vi "CheckCore.vi"(8 "error in (no error)":errorcluster, 9 "# of Refs":i32, 10 "References":refnum<vi>[](array[refnum]), 11 "Invoke in":refnum<class "Invoke.lvclass">) -> (0 "error out":errorcluster, 1 "Reject?":bool, 2 "dup References":refnum<vi>[](array[refnum]), 3 "Invoke out":refnum<class "Invoke.lvclass">)   [LabVIEW 2014, in "BuildSecurity.lvlib" / "Invoke.lvclass"]
doc: "Determines if any blacklisted invoke node exists in the VI."
uses:
  Invoke.lvclass
  Blacklist.lvclass/Blacklist.ctl
  ReadItems.vi
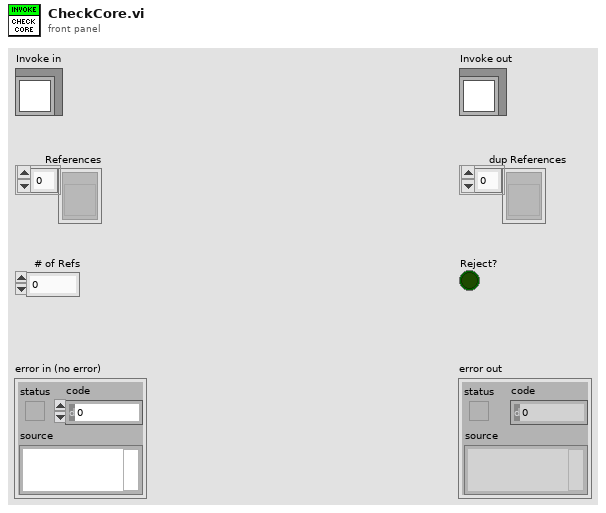
[diagram p1: front panel]
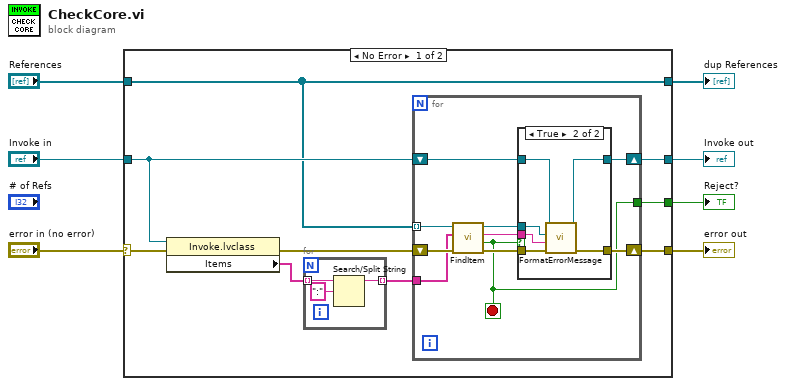
[diagram p0: block diagram]
diagram:
  n1 = case shown="No Error" "error in (no error)" {
    selector: "error in (no error)" -> [w16 w40]
    tunnel: "Invoke in" -> [w13 w39]
    tunnel: [w10 w40] -> w5
    tunnel: [w9 w39] -> w4
    tunnel: "References" -> [w11 w38]
    tunnel: [w11 w38] -> w2
    tunnel: [w8 _] -> w1
    frame No Error {
      n2 = property class="Invoke.lvclass"(reference=w13, error in=w16) -> (error out=w12:errorcluster, "Items"=w15:string[])  [unwired: 1 out]
      n3 = for {
        tunnel: w15 -> [w37] mode=indexing
        tunnel: [w35] -> w14 mode=indexing
        n4 = Search/Split String(string=w37, search string/char (-)=":") -> (substring before match=w35:string)  [unwired: 1 in, 2 out]
      }
      n5 = for {
        tunnel: w14 -> [w25]
        shift-right: [w22] -> w10
        shift-left: w12 -> [w26]
        shift-right: [w20] -> w9
        shift-left: w13 -> [w21]
        tunnel: w11 -> [w24] mode=indexing
        tunnel: [w17] -> w8
        stop <- w17 stop-if-true
        n6 = call "FindItem.vi"("error in"=w26, "Items"=w25, "GObj Refnum"=w24) -> ("error out"=w23:errorcluster, "Reject?"=w17:bool, "Identifier"=w18:string, "dup GObj Refnum"=w19:refnum<vi>)  [unwired: 5 in]
        n7 = case shown="True" w17 {
          tunnel: w23 -> [w28 w34]
          tunnel: [w28 w33] -> w22
          tunnel: w21 -> [w27 w32]
          tunnel: [w27 w31] -> w20
          tunnel: w19 -> [_ w30]
          tunnel: w18 -> [_ w29]
          frame False {
          }
          frame True {
            n8 = call-dynamic "FormatErrorMessage.vi"("error in (no error)"=w34, "Node qualifier"=w29, "GObj Refnum"=w30, "Blacklist in"=w32) -> ("error out"=w33:errorcluster, "Blacklist out"=w31:refnum<class "Invoke.lvclass">)  [unwired: 5 in, 1 out]
          }
        }
      }
    }
    frame Error {
    }
  }
  "error out" <- w5
  "Invoke out" <- w4
  "dup References" <- w2
  "Reject?" <- w1
